vi "Execute.vi"(8 "error in (no error)":errorcluster, 10 "Context in":refnum<class "Context.lvclass">, 11 "Start Scan Command in":refnum<class "Start Testing Command.lvclass">) -> (0 "error out":errorcluster, 2 "Context out":refnum<class "Context.lvclass">, 3 "Start Scan Command out":refnum<class "Start Testing Command.lvclass">)   [LabVIEW 2015, in "Start Testing Command.lvclass"]
uses:
  Start Testing Command.lvclass
  Context/Context.lvclass
  Start Testing Command.lvclass/Start Testing Command.ctl
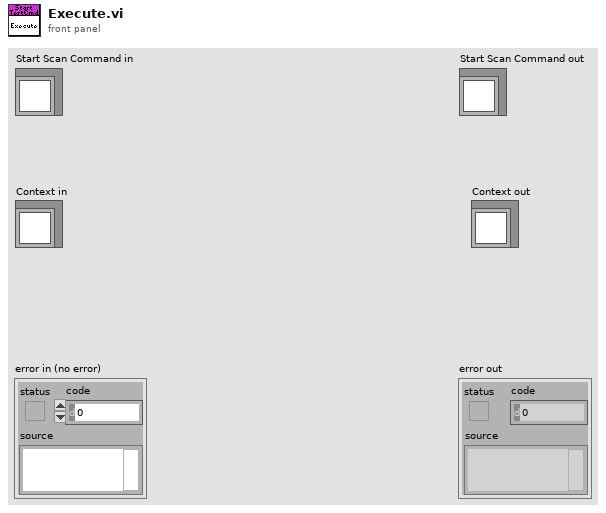
[diagram p1: front panel]
types:
  T1 = typedef "FAMT Typedefs.lvlib/TestSettings.ctl" = cluster{"Operator":string, "Notes":string, "Actuator Serial Number":string, "Test Stand Serial Number":string, "Axial Load Cell Sensitivity":dbl, "Lateral Load Cell Sensitivity":dbl, "Actuator Type":T2}
  T2 = typedef "RTFAILC.lvlib/FATypes.ctl" = enum16{"SingleAxis", "LateralDualAxis", "CrossLateralDualAxis"}
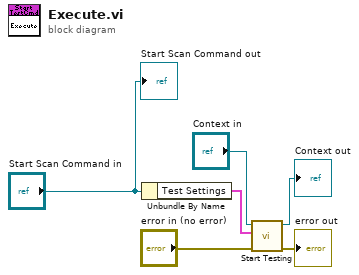
[diagram p0: block diagram]
diagram:
  n1 = Unbundle By Name("Start Scan Command in") -> ("Test Settings"=w3:T1)
  n2 = call "Start Testing.vi"("error in (no error)"="error in (no error)", "Test Settings"=w3, "Context in"="Context in") -> ("error out"=→"error out":errorcluster, "Context out"=→"Context out":refnum<class "Context.lvclass">)  [unwired: 7 in]
  "Start Scan Command out" <- "Start Scan Command in"
